vi "Show Panel.vi"(8 "Value":variant, 9 "Datum Name":string, 10 "Show Panel Boolean":string, 11 "VI in":refnum<vi>) -> ()   [LabVIEW 2017, in "ListboxBusMonitor.lvlib" / "ListboxBusMonitorPanel.lvclass"]
uses:
  ListboxBusMonitorPanel.lvclass
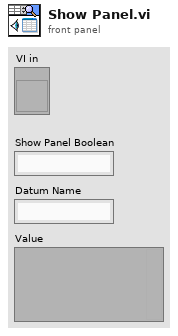
[diagram p1: front panel]
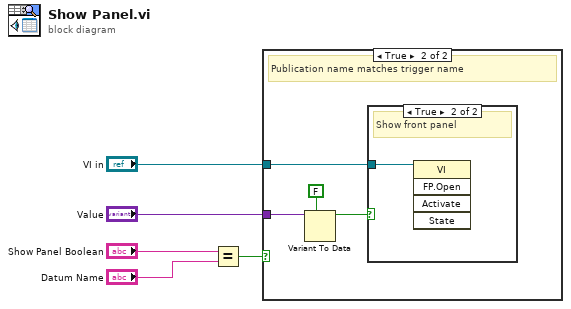
[diagram p0: block diagram]
diagram:
  n1 = Equal?(x="Show Panel Boolean", y="Datum Name") -> (x = y?=w3:bool)
  n2 = case shown="True" w3 {
    tunnel: "Value" -> [_ w9]
    tunnel: "VI in" -> [_ w6]
    frame False {
    }
    frame True {
      # "Publication name matches trigger name"
      n3 = Variant To Data(type=FALSE, Variant=w9) -> (data=w7:bool)  [unwired: 1 in, 1 out]
      n4 = case shown="True" w7 {
        tunnel: w6 -> [_ w10]
        frame False {
          # "Don't do anything"
        }
        frame True {
          # "Show front panel"
          n5 = invoke class="VI" method="FP.Open"(reference=w10) -> ()  [unwired: 4 in, 5 out]
        }
      }
    }
  }
